vi "Read from FIFO.vi"() -> (1 "Time Out?":bool, 2 "Element":u8, 3 "Array":u8[](array[numeric]))   [LabVIEW 2014]
uses:
  <vilib>/rvi/interface/RandomDataEmulation/niFpgaRandomDataHandleErrors.vi
  <vilib>/rvi/DataTransferAndStorage/Container/XNode/niFpgaContainer.xnode
  <vilib>/rvi/interface/RandomDataEmulation/nirviRandomDataFpgaReadWriteTemplate.vi
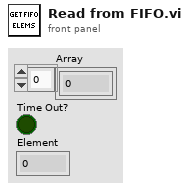
[diagram p1: front panel]
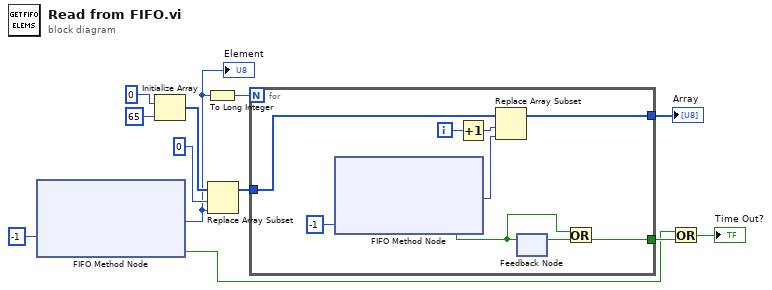
[diagram p0: block diagram]
diagram:
  n1 = xnode ("FIFO Method Node")("Timeout"=-1) -> ("Element"=w5:u8, "Timed Out?"=w1:bool)  [unwired: 1 in, 1 out]
  "Element" <- w5
  n2 = Initialize Array(u8 0 ("Timeout"), 65 ("dimension size")) -> (w10:u8[])
  n3 = To Long Integer(number=w5) -> (32bit integer=w4:i32)
  n4 = Replace Array Subset(array=w10, new element=w5, index=0) -> (w7:u8[])
  n5 = for {
    N: w4 -> [_]
    tunnel: w7 -> [w21]
    tunnel: [w16] -> w6
    tunnel: [w14] -> w3
    i -> [w20]
    n6 = xnode ("FIFO Method Node")("Timeout"=-1) -> ("Element"=w18:u8, "Timed Out?"=w13:bool)  [unwired: 1 in, 1 out]
    n7 = Increment(x=w20) -> (x+1=w19:i32)
    n8 = Replace Array Subset(array=w21, new element=w18, index=w19) -> (w16:u8[])
    n9 = feedback-in #1(w13) -> ()
    n10 = feedback #1() -> (w15:bool)  [unwired: 1 in]
    n11 = Or(x=w13, y=w15) -> (x .or. y?=w14:bool)
  }
  "Array" <- w6
  n12 = Or(x=w1, y=w3) -> (x .or. y?=→"Time Out?":bool)
